vi "AdaptToInputs.vi"(0 "XRef":T10, 1 "Term Types":T7, 2 "State In":T1) -> (14 "Reply":T5, 15 "Fatal Error Out":T4, 16 "State Out":T1)   [LabVIEW 2021, in "FirstXNode .xnode"]
uses:
  FirstXNode .xnode
  <vilib>/XNodeSupport/XNodeXNodeRef.ctl
  <vilib>/XNodeSupport/XNodeTermTypeIDPairs.ctl
  <vilib>/XNodeSupport/XNodeTermTypeIDPair.ctl
  <vilib>/XNodeSupport/XNodeType.ctl
  <vilib>/XNodeSupport/XNodeString.ctl
  State.ctl
  <vilib>/XNodeSupport/XNodeBounds.ctl
  <vilib>/XNodeSupport/XNodeInt.ctl
  <vilib>/XNodeSupport/XNodeStringArray.ctl
  <vilib>/XNodeSupport/XNodeErrorCluster.ctl
  <vilib>/XNodeSupport/NI_XNodeSupport.lvlib
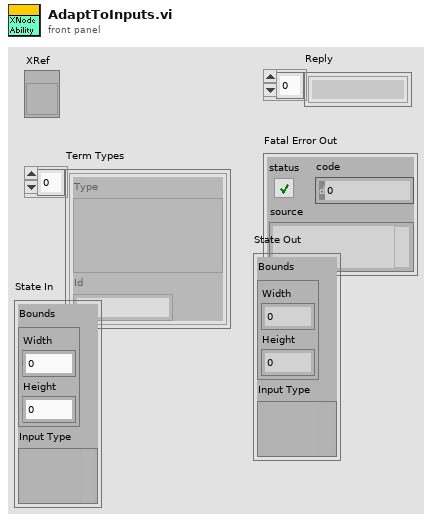
[diagram p1: front panel]
types:
  T1 = typedef "FirstXNode .xnode/State.ctl" = cluster{"Bounds":T2, "Input Type":variant}
  T2 = typedef "NI_XNodeSupport.lvlib/XNodeBounds.ctl" = cluster{"Width":T3, "Height":T3}
  T3 = typedef "NI_XNodeSupport.lvlib/XNodeInt.ctl" = i32
  T4 = typedef "NI_XNodeSupport.lvlib/XNodeErrorCluster.ctl" = errorcluster
  T5 = typedef "NI_XNodeSupport.lvlib/XNodeStringArray.ctl" = T6[]
  T6 = typedef "NI_XNodeSupport.lvlib/XNodeString.ctl" = string
  T7 = typedef "NI_XNodeSupport.lvlib/XNodeTermTypeIDPairs.ctl" = T8[]
  T8 = typedef "NI_XNodeSupport.lvlib/XNodeTermTypeIDPair.ctl" = cluster{"Type":T9, "Id":T6}
  T9 = typedef "NI_XNodeSupport.lvlib/XNodeType.ctl" = variant
  T10 = typedef "NI_XNodeSupport.lvlib/XNodeXNodeRef.ctl" = refnum<vi>
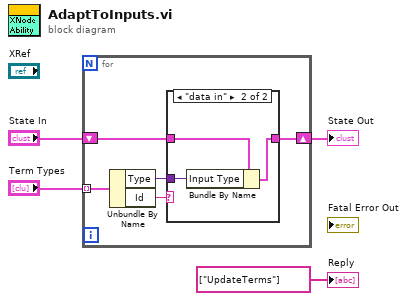
[diagram p0: block diagram]
diagram:
  n1 = for {
    tunnel: "Term Types" -> [w9] mode=indexing
    shift-right: [w5] -> w2
    shift-left: "State In" -> [w6]
    n2 = Unbundle By Name(w9) -> ("Type"=w7:T9, "Id"=w8:T6)
    n3 = case shown="\"data in\"" w8 {
      tunnel: w7 -> [_ w11]
      tunnel: w6 -> [w10 w13]
      tunnel: [w10 w12] -> w5
      frame "", Default {
      }
      frame "data in" {
        n4 = Bundle By Name(cluster=w13, "Input Type"=w11) -> (w12:T1)
      }
    }
  }
  "State Out" <- w2
  "Reply" <- T5 ["UpdateTerms"] ("Reply")
